vi "select rates simple.vi"(9 "method in":T1={"sampling interval"=0.1, "samples to average"=1, "data interval"=0.0, "stream data"=FALSE, "file path"=refnum, "command"={"command"=enum."Idle", "start time (ms)"=0, "Channel Indices"=[], "Scans per Sample"=1}} {"command"."Scans per Sample" min=1; "data interval" format="%.2f"; "samples to average" min=1 step=1; "sampling interval" format="%.2f"}) -> (3 "method out":T1={"sampling interval"=0.1, "samples to average"=1, "data interval"=0.0, "stream data"=FALSE, "file path"=refnum, "command"={"command"=enum."Idle", "start time (ms)"=0, "Channel Indices"=[], "Scans per Sample"=1}} {"command"."Scans per Sample" min=1; "data interval" format="%.2f"; "samples to average" min=1 step=1; "sampling interval" format="%.2f"}, 8 "new samples to average":u32=1 min=1 step=1, 10 "new data interval":sgl format="%.5f", 13 "canceled":bool)   [LabVIEW 2010]
uses:
  DAC apps/support/method.ctl
  DataServer/command cluster.ctl
  DataServer/command.ctl
  DataServer/Server Stats.vi
panel:
  in  "Data frequency":ext=1.0 format="%.2f"
  out "Maximum data frequency":dbl format="%.2f"
  in  "cancel":bool
  in  "ok":bool
  # "hz"
  # "hz"
  # "s"
  # "s"
  # "s"
  # "s"
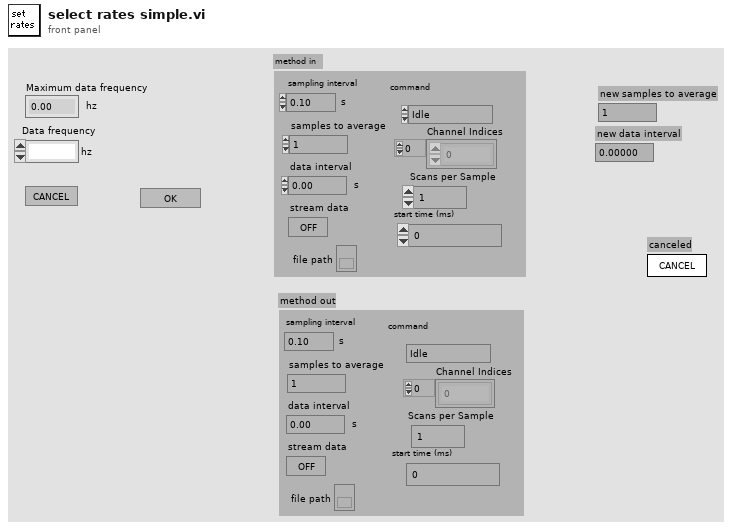
[diagram p1: front panel]
types:
  T1 = typedef "method.ctl" = cluster{"sampling interval":sgl, "samples to average":u32, "data interval":sgl, "stream data":bool, "file path":refnum<file>, "command":T2}
  T2 = typedef "command cluster.ctl" = cluster{"command":T3, "start time (ms)":u32, "Channel Indices":i32[], "Scans per Sample":i32}
  T3 = typedef "command.ctl" = enum16{"Idle", "Send Data", "Send 1 Scan", "Logoff"}
  T4 = typedef "Server stats.ctl" = cluster{"scan rate":dbl, "# connections":i32, "channel settings":cluster{"Name":string, "upper input limits":sgl, "lower input limits":sgl, "Location":string}[]}
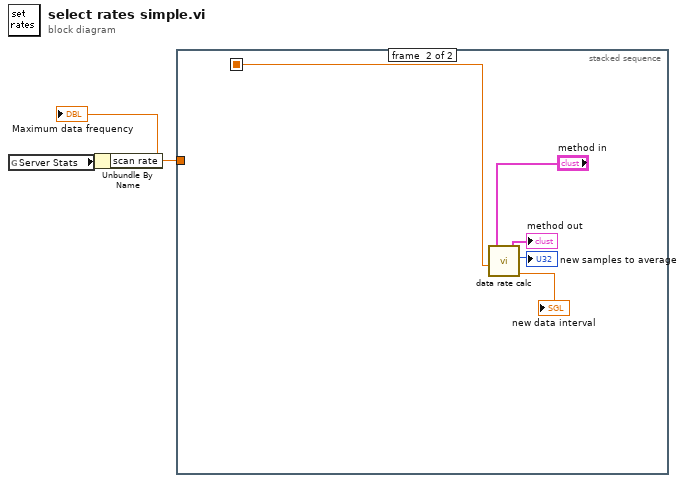
[diagram p0: block diagram]
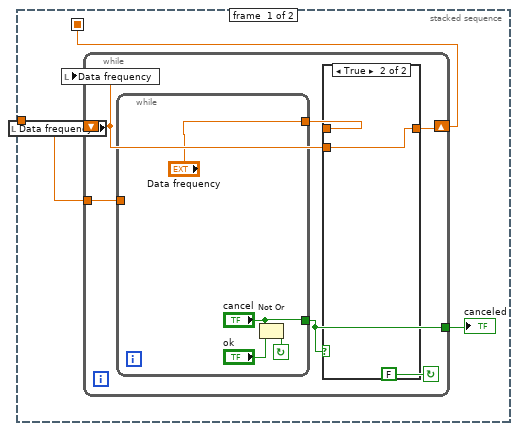
[diagram p2: hidden frame]
diagram:
  n1 = global read "Server Stats.vi" "Server Stats"() -> (w1:T4)
  n2 = Unbundle By Name(w1) -> ("scan rate"=w2:dbl)
  "Maximum data frequency" <- w2
  n3 = stacked-sequence {
    seq-local: [w6 _] -> [_ w22]
    tunnel: w2 -> [w3 _]
    frame #0 {
      n4 = local read "Data frequency"() -> (w4:ext)
      n5 = while {
        tunnel: w3 -> [w8]
        tunnel: [w9] -> w5
        shift-left: w4 -> [w12]
        shift-right: [w11] -> w6
        stop <- FALSE continue-if-true
        n6 = local write "Data frequency"(w12) -> ()
        n7 = while {
          tunnel: w8 -> [_]
          tunnel: ["cancel"] -> w9
          tunnel: ["Data frequency"] -> w10
          stop <- w15 continue-if-true
          n8 = Not Or(1:"ok", 2:"cancel") -> (0:w15:bool)
        }
        n9 = case shown="True" w9 {
          tunnel: [w17 w18] -> w11
          tunnel: w10 -> [w17 _]
          tunnel: w12 -> [_ w18]
          frame False {
          }
          frame True {
          }
        }
      }
      "canceled" <- w5
    }
    frame #1 {
      n10 = call "data rate calc.vi"("Data frequency"=w22, "method in"="method in") -> ("new data interval"=→"new data interval":sgl, "new samples to average"=→"new samples to average":u32, "method out"=→"method out":T1)  [unwired: 2 in, 1 out]
    }
  }
